vi "oa_Trigger Single Channel Signal.vi"(6 "block size":i32=1024, 7 "history signal":dbl[](array[numeric]), 8 "trigger period [rev]":dbl=1.0, 9 "dr":dbl=1.0, 10 "history r0":dbl=1.0, 11 "signal to be triggered":dbl[](array[numeric])) -> (0 "dr out":dbl=1.0, 1 "triggered signal":dbl[](array[numeric]), 2 "triggered r0":dbl=1.0, 3 "history r0":dbl, 5 "history signal out":dbl[](array[numeric]))   [LabVIEW 2017, in "SoundVib_OAUtility.lvlib"]
uses:
  <vilib>/addons/Sound and Vibration/Order Analysis/Utility/SoundVib_OAUtility.lvlib
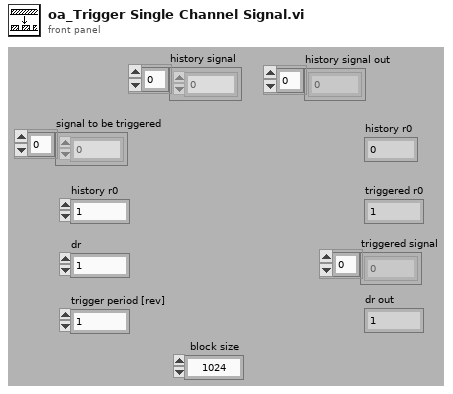
[diagram p1: front panel]
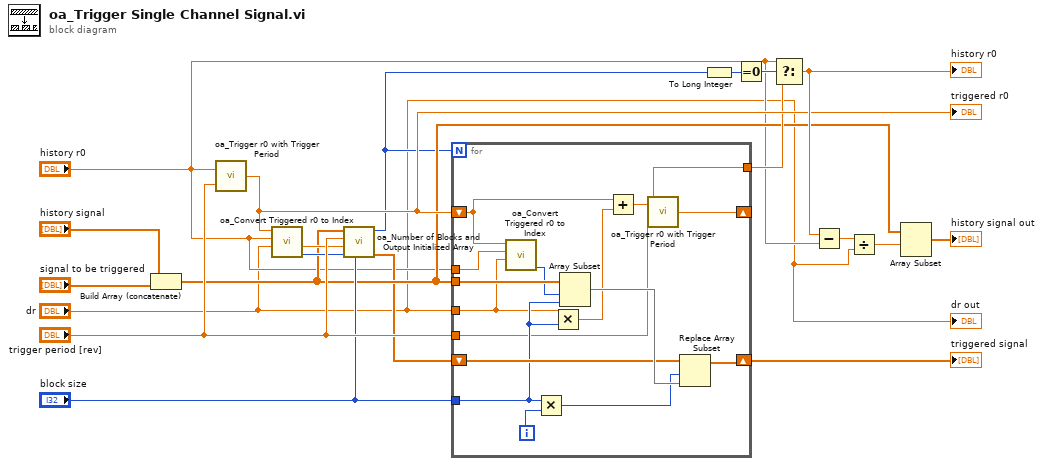
[diagram p0: block diagram]
diagram:
  n1 = Build Array (concatenate)("history signal", "signal to be triggered") -> (w9:dbl[])
  n2 = call <vilib>:"oa_Trigger r0 with Trigger Period.vi"("trigger period [rev]"="trigger period [rev]", "r0"="history r0") -> ("triggered r0"=w14:dbl)
  "triggered r0" <- w14
  n3 = call <vilib>:"oa_Convert Triggered r0 to Index.vi"("dr"="dr", "r0"="history r0", "triggered r0"=w14) -> ("index"=w13:i32, "dr out"=w12:dbl)  [unwired: 6 in, 1 out]
  n4 = call <vilib>:"oa_Number of Blocks and Output Initialized Array.vi"("block size"="block size", "index"=w13, "dr"=w12, "trigger period [rev]"="trigger period [rev]", "even angle signal"=w9) -> ("initialized array"=w8:dbl[], "number of blocks"=w7:i32)  [unwired: 5 in]
  n5 = for {
    N: w7 -> [_]
    shift-right: [w31] -> w1
    shift-left: w8 -> [w32]
    tunnel: w9 -> [w28]
    shift-right: [w25] -> _
    shift-left: w14 -> [w24]
    tunnel: "dr" -> [w22]
    tunnel: "block size" -> [w30]
    tunnel: "trigger period [rev]" -> [w26]
    tunnel: "history r0" -> [w23]
    tunnel: [w27] -> w10
    i -> [w35]
    n6 = call <vilib>:"oa_Convert Triggered r0 to Index.vi"("dr"=w22, "r0"=w23, "triggered r0"=w24) -> ("index"=w21:i32)  [unwired: 6 in, 2 out]
    n7 = Multiply(x=w30, y=w35) -> (x*y=w33:i32)
    n8 = Multiply(x=w22, y=w30) -> (x*y=w29:dbl)
    n9 = Array Subset(array=w28, index=w21, length=w30) -> (w34:dbl[])
    n10 = Add(x=w24, y=w29) -> (x+y=w27:dbl)
    n11 = call <vilib>:"oa_Trigger r0 with Trigger Period.vi"("trigger period [rev]"=w26, "r0"=w27) -> ("triggered r0"=w25:dbl)
    n12 = Replace Array Subset(array=w32, new element=w34, index=w33) -> (w31:dbl[])
  }
  "triggered signal" <- w1
  n13 = To Long Integer(number=w7) -> (32bit integer=w18:i32)
  n14 = Equal To 0?(x=w18) -> (x = 0?=w17:bool)
  n15 = Select(t="history r0", s=w17, f=w10) -> (s? t:f=w16:dbl)
  "history r0" <- w16
  n16 = Subtract(x=w16, y="history r0") -> (x-y=w20:dbl)
  n17 = Divide(x=w20, y="dr") -> (x/y=w19:dbl)
  n18 = Array Subset(array=w9, index=w19) -> (→"history signal out":dbl[])  [unwired: 1 in]
  "dr out" <- "dr"
